vi "TL2100EXAM01_Q18.vi"() -> ()   [LabVIEW 2020]
panel:
  out "Possible eye damage":bool
  out "Lumens":dbl(slide) scale=0.0..1500.0 scale format="%.2f"
  out "Sensor Volts":dbl(slide) scale=0.0..5.0 scale format="%.2f"
  in  "stop":bool
  out "SCC Volts":dbl(slide) scale=-10.0..10.0 scale format="%.2f"
  out "AtoD In":i16 format="%04x"
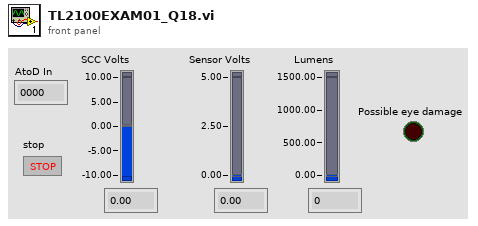
[diagram p1: front panel]
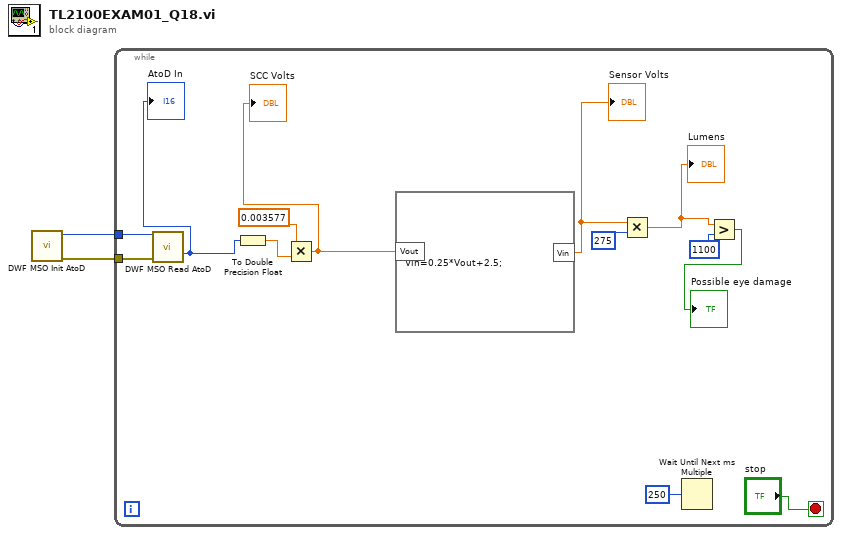
[diagram p0: block diagram]
diagram:
  n1 = call "DWF MSO Init AtoD.vi"() -> ("Error Out"=w1:errorcluster, "Instrument Handle Out"=w2:u32)  [unwired: 10 in]
  n2 = while {
    tunnel: w2 -> [w14]
    tunnel: w1 -> [w13]
    stop <- "stop" stop-if-true
    n3 = call "DWF MSO Read AtoD.vi"("Instrument Handle In AtoD"=w14, "Error In"=w13) -> ("AtoD"=w11:i16)  [unwired: 12 in, 1 out]
    "AtoD In" <- w11
    n4 = To Double Precision Float(number=w11) -> (double precision float=w10:dbl)
    n5 = Multiply(x=0.003577, y=w10) -> (x*y=w8:dbl)
    "SCC Volts" <- w8
    n6 = formula code="Vin=0.25*Vout+2.5;"("Vout"=w8) -> ("Vin"=w6:dbl)
    "Sensor Volts" <- w6
    n7 = Multiply(x=w6, y=275) -> (x*y=w4:dbl)
    "Lumens" <- w4
    n8 = Wait Until Next ms Multiple(millisecond multiple=250) -> ()  [unwired: 1 out]
    n9 = Greater?(x=w4, y=1100) -> (0:→"Possible eye damage":bool)
  }
